vi "Read Attributes.vi"(11 "Set ForecastData Long Msg":refnum<class "Set ForecastData Long Msg.lvclass">) -> (2 "Payload":cluster{"ForecastData":T1})   [LabVIEW 2018, in "Device Communication and Control Abstract Actor.lvlib" / "Set ForecastData Long Msg.lvclass"]
uses:
  Set ForecastData Long Msg.lvclass
  <vilib>/ORNL/CSEISMIC DDS/CSEISMIC DDS Base/Data Types/ForecastData_Data.ctl
  <vilib>/ORNL/CSEISMIC DDS/CSEISMIC DDS Base/Data Types/Controls/DeviceID.ctl
  Set ForecastData Long Msg.lvclass/Set ForecastData Long Msg.ctl
  <vilib>/ORNL/CSEISMIC DDS/CSEISMIC DDS Base/CSEISMIC DDS.lvclass
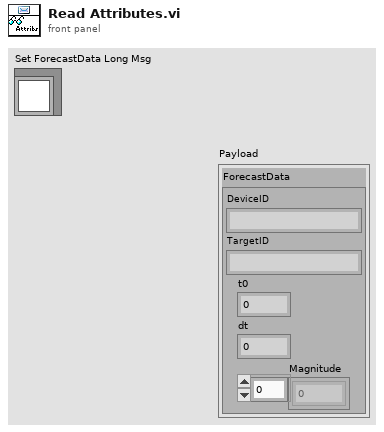
[diagram p1: front panel]
types:
  T1 = typedef "CSEISMIC DDS.lvlib/CSEISMIC DDS.lvclass/ForecastData_Data.ctl" = cluster{"DeviceID":T2, "TargetID":T2, "t0":dbl, "dt":dbl, "Magnitude":dbl[]}
  T2 = typedef "CSEISMIC DDS.lvlib/CSEISMIC DDS.lvclass/DeviceID.ctl" = string
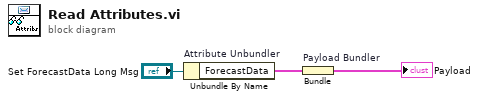
[diagram p0: block diagram]
diagram:
  n1 = Unbundle By Name "Attribute Unbundler"("Set ForecastData Long Msg") -> ("ForecastData"=w1:T1)
  n2 = Bundle "Payload Bundler"("ForecastData"=w1) -> (→"Payload":cluster{"ForecastData":T1})  [unwired: 1 in]
